vi "Taikoi_GetSystemStatus.vi"(8 "error in (no error)":errorcluster, 10 "LBSysStatRef":refnum<vi>, 11 "USBIdx":i32) -> (0 "error out":errorcluster, 1 "QError":bool, 2 "needUpdate":bool, 3 "Status":string)   [LabVIEW 2010]
uses:
  _lib/PDLM/pdlm_lib_x86_x64_UIThread.llb/PDLM_NamedBit.ctl
  _lib/PDLM/pdlm_lib_x86_x64_UIThread.llb/PDLM_Status.ctl
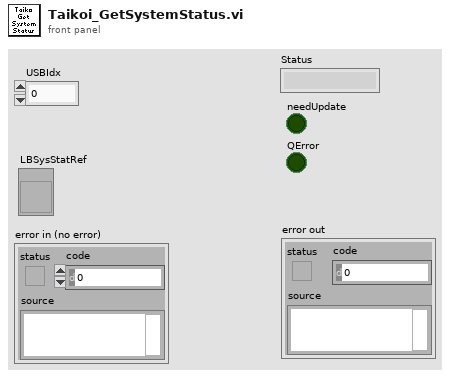
[diagram p1: front panel]
types:
  T1 = typedef "PDLM_Status.ctl" = T2[]
  T2 = typedef "PDLM_NamedBit.ctl" = cluster{"StatName":string, "StatBit":bool}
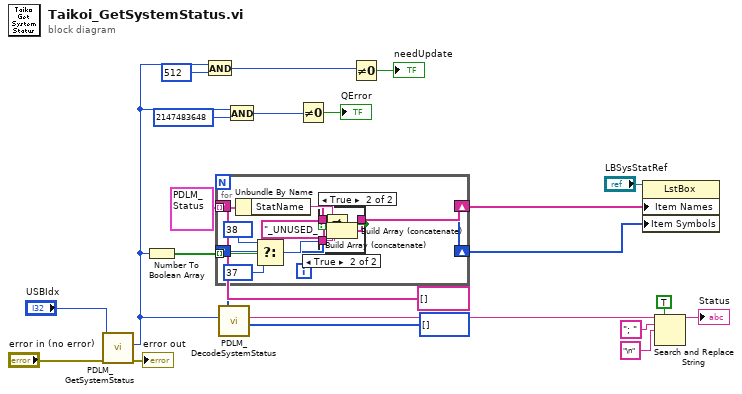
[diagram p0: block diagram]
diagram:
  n1 = call "PDLM_GetSystemStatus.vi"("error in (no error)"="error in (no error)", "USBIdx"="USBIdx") -> ("error out"=→"error out":errorcluster, "state"=w5:u32)  [unwired: 7 in, 1 out]
  n2 = Number To Boolean Array(number=w5) -> (Boolean array=w19:bool[])
  n3 = And(x=w5, y=u32 512) -> (x .and. y?=w8:u32)
  n4 = for {
    tunnel: w19 -> [w33] mode=indexing
    tunnel: T1 [{"StatName"="INITIALIZING", "StatBit"=FALSE}, {"StatName"="DEVICE_UNCALIBRATED", "StatBit"=FALSE}, {"StatName"="COMMISSIONING_MODE", "StatBit"=FALSE}, {"StatName"="LASERHEAD_SAFETY_MODE", "StatBit"=FALSE}, {"StatName"="FW_UPDATE_RUNNING", "StatBit"=FALSE}, {"StatName"="DEVICE_DEFECT", "StatBit"=FALSE}, {"StatName"="DEVICE_INCOMPATIBLE", "StatBit"=FALSE}, {"StatName"="BUSY", "StatBit"=FALSE}, {"StatName"="EXCLUSIVE_SW_OP_GRANTED", "StatBit"=FALSE}, {"StatName"="PARAMETER_CHANGES_PENDING", "StatBit"=FALSE}, {"StatName"="_UNUSED_", "StatBit"=FALSE}, {"StatName"="LASERHEAD_CHANGED", "StatBit"=FALSE}, {"StatName"="LASERHEAD_MISSING", "StatBit"=FALSE}, {"StatName"="LASERHEAD_DEFECT", "StatBit"=FALSE}, {"StatName"="LASERHEAD_UNKNOWN_TYPE", "StatBit"=FALSE}, {"StatName"="LASERHEAD_DECALIBRATED", "StatBit"=FALSE}, {"StatName"="LASERHEAD_DIODE_TEMP_TOO_LOW", "StatBit"=FALSE}, {"StatName"="LASERHEAD_DIODE_TEMP_TOO_HIGH", "StatBit"=FALSE}, {"StatName"="LASERHEAD_DIODE_OVERHEATING", "StatBit"=FALSE}, {"StatName"="LASERHEAD_CASE_OVERHEATING", "StatBit"=FALSE}, {"StatName"="LASERHEAD_FAN_RUNNING", "StatBit"=FALSE}, {"StatName"="LASERHEAD_INCOMPATIBLE", "StatBit"=FALSE}, {"StatName"="LOCKED_BY_EXPIRED_DEMO_MODE", "StatBit"=FALSE}, {"StatName"="LOCKED_BY_ON_OFF_BUTTON", "StatBit"=FALSE}, {"StatName"="SOFTLOCK", "StatBit"=FALSE}, {"StatName"="KEYLOCK", "StatBit"=FALSE}, {"StatName"="LOCKED_BY_SECURITY_POLICY", "StatBit"=FALSE}, {"StatName"="INTERLOCK", "StatBit"=FALSE}, {"StatName"="LASERHEAD_PULSE_POWER_INACCURATE", "StatBit"=FALSE}, {"StatName"="_UNUSED_", "StatBit"=FALSE}, {"StatName"="_UNUSED_", "StatBit"=FALSE}, {"StatName"="ERRORMSG_PENDING", "StatBit"=FALSE}] ("Status") -> [w34] mode=indexing
    shift-right: [w25] -> w20
    shift-left: string[] [] ("Array") -> [w26]
    shift-right: [w23] -> w21
    shift-left: i32[] [] ("Array") -> [w24]
    n5 = Unbundle By Name(w34) -> ("StatName"=w27:string)
    n6 = Select(t=38, s=w33, f=37) -> (s? t:f=w30:i32)
    n7 = Not Equal?(x=w27, y="_UNUSED_") -> (x != y?=w28:bool)
    n8 = case shown="True" w28 {
      tunnel: w24 -> [w35 w37]
      tunnel: w30 -> [_ w36]
      tunnel: [w35 w38] -> w23
      frame False {
      }
      frame True {
        n9 = Build Array (concatenate)(w37, w36) -> (w38:i32[])
      }
    }
    n10 = case shown="True" w28 {
      tunnel: w26 -> [w39 w41]
      tunnel: w27 -> [_ w40]
      tunnel: [w39 w42] -> w25
      frame False {
      }
      frame True {
        n11 = Build Array (concatenate)(w41, w40) -> (w42:string[])
      }
    }
  }
  n12 = call "PDLM_DecodeSystemStatus.vi"("state"=w5) -> ("Buffer"=w13:string)  [unwired: 8 in, 2 out]
  n13 = And(x=w5, y=u32 2147483648) -> (x .and. y?=w4:u32)
  n14 = Not Equal To 0?(x=w4) -> (x != 0?=→"QError":bool)
  n15 = Not Equal To 0?(x=w8) -> (x != 0?=→"needUpdate":bool)
  n16 = property class="LstBox"(reference="LBSysStatRef", "Item Names"=w20, "Item Symbols"=w21) -> ()  [unwired: 1 in, 2 out]
  n17 = Search and Replace String(replace all?=TRUE ("replace all? (F)"), input string=w13, search string="; ", replace string="\n" ("replace string (\"\")")) -> (result string=→"Status":string)  [unwired: 4 in, 3 out]
